vi "Write TDMS Data Objects.vi"(8 "error in (no error)":errorcluster, 10 "TDMS Data Objects":refnum<class "TDMS-Data.lvclass">[](array[class]), 11 "TDMS-Container in":refnum<class "TDMS-Container.lvclass">) -> (0 "error out":errorcluster, 3 "TDMS-Container out":refnum<class "TDMS-Container.lvclass">)   [LabVIEW 2014, in "BNT_TDMS.lvlib" / "TDMS-Container.lvclass"]
uses:
  TDMS-Container.lvclass
  TDMSData/TDMS-Data.lvclass
  TDMS-Container.lvclass/TDMS-Container.ctl
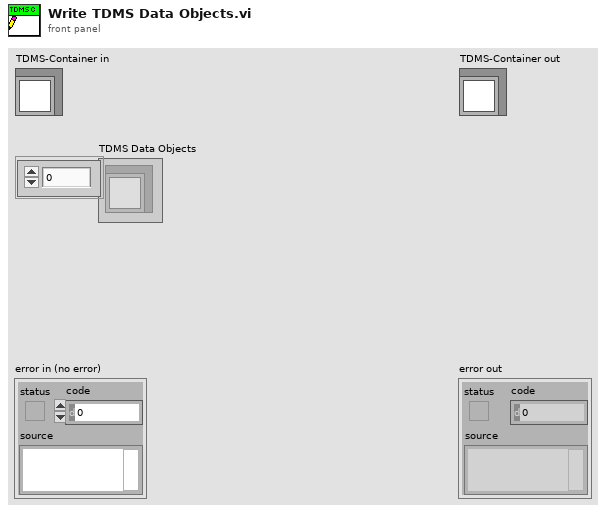
[diagram p1: front panel]
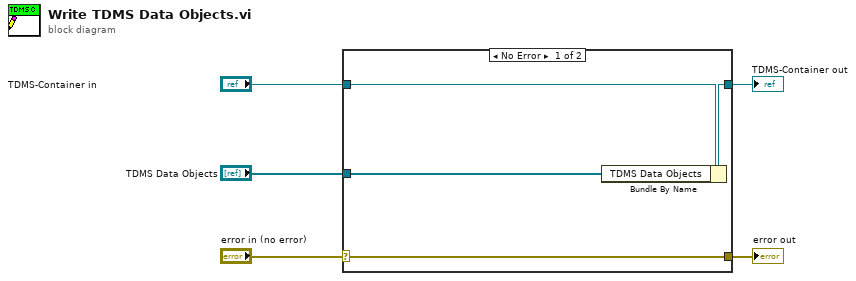
[diagram p0: block diagram]
diagram:
  n1 = case shown="No Error" "error in (no error)" {
    selector: "error in (no error)" -> [w9 w10]
    tunnel: [w9 w10] -> w4
    tunnel: [w7 w11] -> w2
    tunnel: "TDMS-Container in" -> [w8 w11]
    tunnel: "TDMS Data Objects" -> [w6 _]
    frame No Error {
      n2 = Bundle By Name(cluster=w8, "TDMS Data Objects"=w6) -> (w7:refnum<class "TDMS-Container.lvclass">)
    }
    frame Error {
    }
  }
  "error out" <- w4
  "TDMS-Container out" <- w2
